vi "Control WavePond.vi"(8 "Error In":errorcluster, 9 "Parameter":string, 10 "Command":T1(ring)) -> (0 "Error Out":errorcluster, 2 "Return Message":string, 3 "standard output":string)   [LabVIEW 2014]
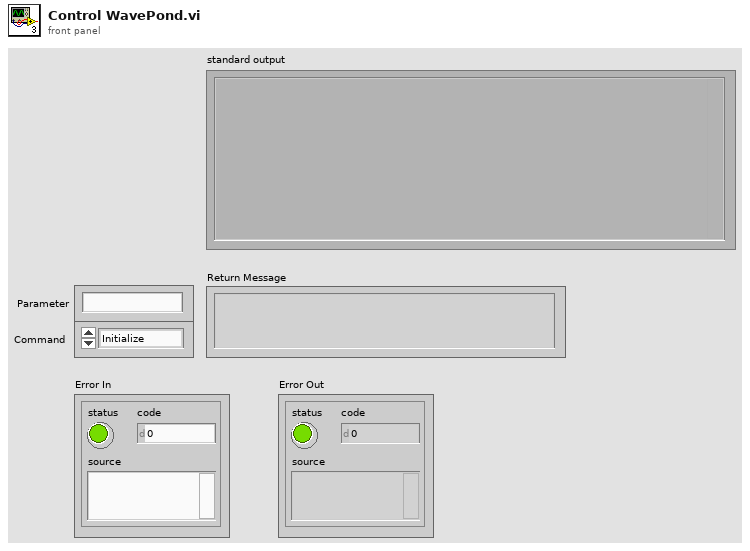
[diagram p1: front panel]
types:
  T1 = enum16{"Initialize", "SetFrequency", "SetAtten", "WriteData", "EnableSweep", "SetLoopCnt", "SetClkDiv", "SelExtTrig", "SoftTrig", "En_SqWave"}
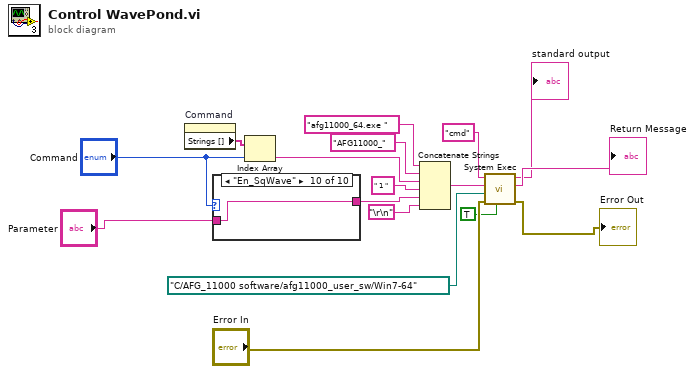
[diagram p0: block diagram]
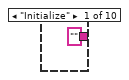
[diagram p2: hidden frame]
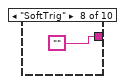
[diagram p9: hidden frame]
diagram:
  n1 = property on="Command" class="Enum (strict)"() -> ("Strings []"=w9:string[])  [unwired: 2 in, 2 out]
  n2 = case shown="\"En_SqWave\"" "Command" {
    tunnel: ["" ("Parameter") w19 w20 w21 w22 w23 w24 "" w26 w27] -> w11
    tunnel: "Parameter" -> [_ w19 w20 w21 w22 w23 w24 _ w26 w27]
    frame "Initialize" {
    }
    frame "SetFrequency" {
    }
    frame "SetAtten" {
    }
    frame "WriteData" {
    }
    frame "EnableSweep" {
    }
    frame "SetLoopCnt" {
    }
    frame "SetClkDiv" {
    }
    frame "SoftTrig" {
    }
    frame "SelExtTrig" {
    }
    frame "En_SqWave" {
    }
  }
  n3 = Index Array(array=w9, index="Command") -> (element=w8:string)
  n4 = Concatenate Strings("afg11000_64.exe " ("string"), "AFG11000_" ("string"), w8, " 1 " ("string"), w11, "\r\n") -> (w10:string)
  n5 = call <vilib>:"System Exec.vi"("run minimized? (F)"=TRUE, "error in (no error)"="Error In", "working directory"=path "C:/AFG_11000 software/afg11000_user_sw/Win7-64", "standard input"=w10, "command line"="cmd") -> ("error out"=→"Error Out":errorcluster, "standard error"=→"Return Message":string, "standard output"=→"standard output":string)  [unwired: 3 in, 1 out]
